vi "Backward.vi"(8 "error in (no error)":errorcluster, 10 "how close":dbl) -> (0 "error out":errorcluster, 2 "Done":bool)   [LabVIEW 2019]
uses:
  Simulated Robot/Simulation SubVIs/Simulation SubVIs.lvlib
panel:
  out "Diff.":dbl
  out "Left":dbl
  out "Right":dbl
  out "Diff. x Z":dbl
  out "Left sonar":dbl
  out "Right sonar":dbl
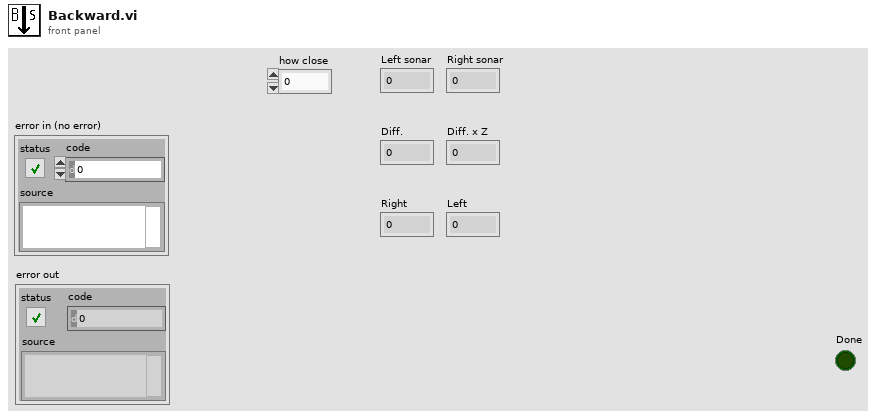
[diagram p1: front panel]
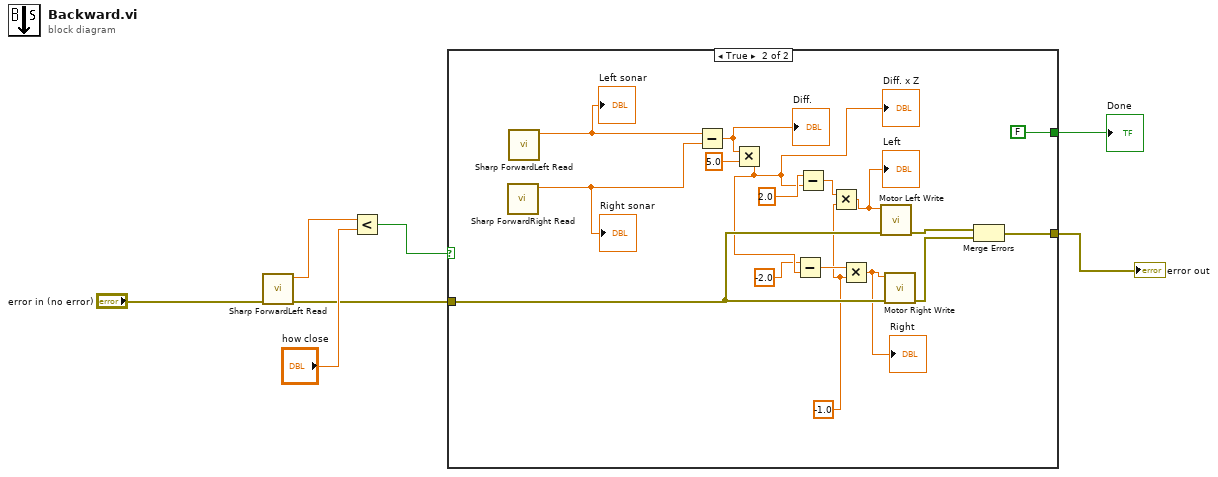
[diagram p0: block diagram]
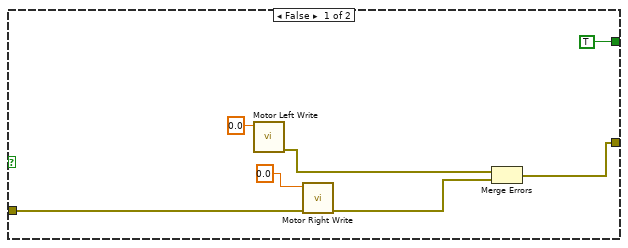
[diagram p2: hidden frame]
diagram:
  n1 = call "Sharp ForwardLeft Read.vi"("error in (no error)"="error in (no error)") -> ("error out"=w1:errorcluster, "ForwardLeft Distance (m)"=w3:dbl)  [unwired: 9 in]
  n2 = Less?(x=w3, y="how close") -> (x < y?=w5:bool)
  n3 = case shown="True" w5 {
    tunnel: [w10 w29] -> w7
    tunnel: w1 -> [w9 w28]
    tunnel: [TRUE ("Done") FALSE ("Done")] -> w4
    frame False {
      n4 = call "Motor Left Write.vi"("left motor ccw velocity (rad/s)"=0.0) -> ("error out"=w14:errorcluster)  [unwired: 10 in]
      n5 = call "Motor Right Write.vi"("error in (no error)"=w9, "right motor ccw velocity (rad/s)"=0.0) -> ("error out"=w13:errorcluster)  [unwired: 9 in]
      n6 = Merge Errors(w14, w13) -> (w10:errorcluster)
    }
    frame True {
      w20 = -1.0
      n7 = call "Sharp ForwardRight Read.vi"() -> ("ForwardRight Distance (m)"=w23:dbl)  [unwired: 10 in, 1 out]
      "Right sonar" <- w23
      n8 = call "Sharp ForwardLeft Read.vi"() -> ("ForwardLeft Distance (m)"=w24:dbl)  [unwired: 10 in, 1 out]
      "Left sonar" <- w24
      n9 = Subtract(x=w24, y=w23) -> (x-y=w27:dbl)
      "Diff." <- w27
      n10 = Multiply(x=w27, y=5.0) -> (x*y=w16:dbl)
      "Diff. x Z" <- w16
      n11 = Subtract(x=-2.0 ("y"), y=w16) -> (x-y=w22:dbl)
      n12 = Subtract(x=2.0 ("left motor ccw velocity (rad/s)"), y=w16) -> (x-y=w21:dbl)
      n13 = Multiply(x=w21, y=w20) -> (x*y=w18:dbl)
      "Left" <- w18
      n14 = Multiply(x=w22, y=w20) -> (x*y=w19:dbl)
      "Right" <- w19
      n15 = call "Motor Left Write.vi"("error in (no error)"=w28, "left motor ccw velocity (rad/s)"=w18) -> ("error out"=w30:errorcluster)  [unwired: 9 in]
      n16 = call "Motor Right Write.vi"("error in (no error)"=w28, "right motor ccw velocity (rad/s)"=w19) -> ("error out"=w31:errorcluster)  [unwired: 9 in]
      n17 = Merge Errors(w30, w31) -> (w29:errorcluster)
    }
  }
  "error out" <- w7
  "Done" <- w4
